vi "Send Stop.vi"(8 "error in (no error)":errorcluster, 11 "Message Queue in":refnum<queue>) -> (0 "error out":errorcluster)   [LabVIEW 2024, in "OOQMH.lvlib" / "Stop.lvclass"]
uses:
  Stop.lvclass
  Message/Message.lvclass
  C:/Users/uspoaotto/OneDrive - Oregon Tool/Desktop/working copies/helperLoop/src/OOQMH/Message/Message.lvclass
  Stop.lvclass/Stop.ctl
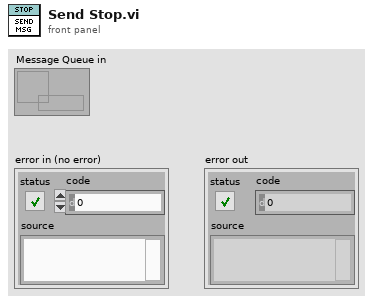
[diagram p1: front panel]
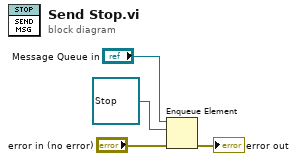
[diagram p0: block diagram]
diagram:
  n1 = Enqueue Element(queue="Message Queue in", element=refnum<class "Stop.lvclass"> refnum ("OOQMH.lvlib:Stop.lvclass"), error in (no error)="error in (no error)") -> (error out=→"error out":errorcluster)  [unwired: 1 in, 2 out]
